vi "FTW-Tree-EditCell.vi"(0 "Tree Ctl Ref":refnum<vi>, 5 "Tag":string, 7 "Column":i32, 11 "error in":errorcluster) -> (4 "Tree Ctl Ref out":refnum<vi>, 15 "error out":errorcluster)   [LabVIEW 2015]
panel:
  # "Inputs"
  # "Outputs"
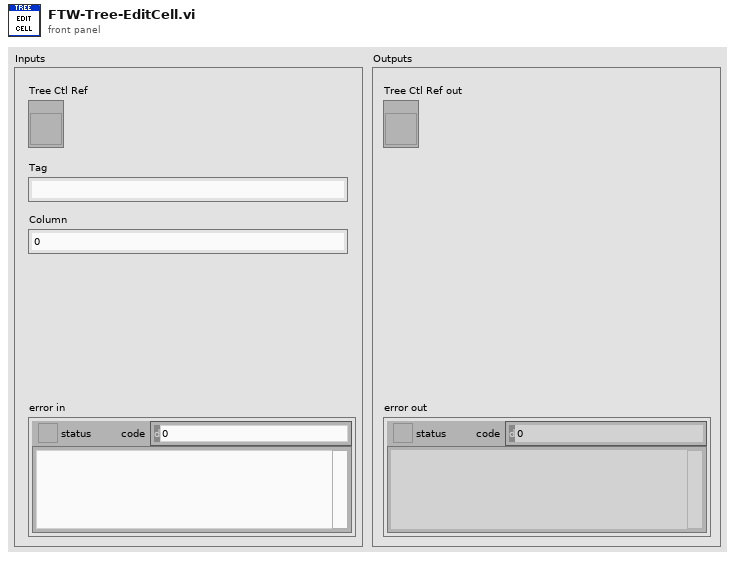
[diagram p1: front panel]
types:
  T1 = cluster{"Active Item Row Number":i32, "Column":i32}
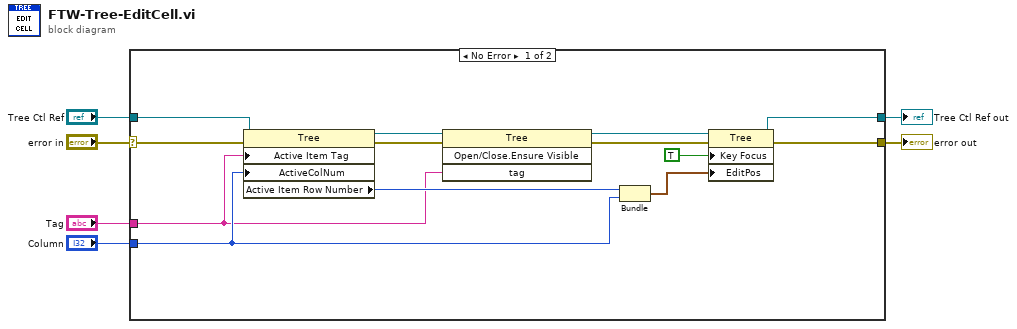
[diagram p0: block diagram]
diagram:
  n1 = case shown="No Error" "error in" {
    selector: "error in" -> [w16 w21]
    tunnel: [w12 w21] -> w6
    tunnel: "Tree Ctl Ref" -> [w15 w20]
    tunnel: "Tag" -> [w7 _]
    tunnel: [w13 w20] -> w3
    tunnel: "Column" -> [w14 _]
    frame No Error {
      n2 = property on="Property Node" class="Tree"(reference=w15, error in=w16, "Active Item Tag"=w7, "ActiveColNum"=w14) -> (reference out=w9:refnum<vi>, error out=w11:errorcluster, "Active Item Row Number"=w18:i32)
      n3 = invoke on="Invoke Node" class="Tree" method="Open/Close.Ensure Visible"(reference=w9, error in=w11, "tag"=w7) -> (reference out=w8:refnum<vi>, error out=w10:errorcluster)  [unwired: 1 in, 2 out]
      n4 = Bundle("Active Item Row Number"=w18, "Column"=w14) -> (w17:T1)  [unwired: 1 in]
      n5 = property on="Property Node" class="Tree"(reference=w8, error in=w10, "Key Focus"=TRUE, "EditPos"=w17) -> (reference out=w13:refnum<vi>, error out=w12:errorcluster)
    }
    frame Error {
    }
  }
  "error out" <- w6
  "Tree Ctl Ref out" <- w3
